vi "ble_wait_ms.vi"(6 "milliseconds to wait (100)":u32=100, 8 "error in (no error)":errorcluster) -> (0 "error out":errorcluster)   [LabVIEW 2017]
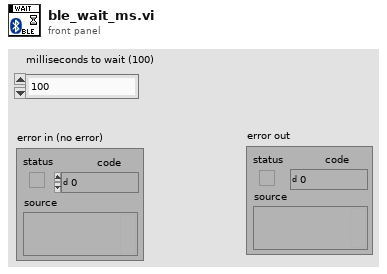
[diagram p1: front panel]
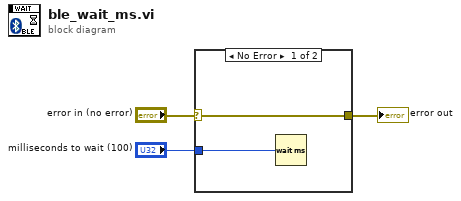
[diagram p0: block diagram]
diagram:
  n1 = case shown="No Error" "error in (no error)" {
    selector: "error in (no error)" -> [w5 w6]
    tunnel: [w5 w6] -> w2
    tunnel: "milliseconds to wait (100)" -> [w4 _]
    frame No Error {
      n2 = Wait (ms)(milliseconds to wait=w4) -> ()  [unwired: 1 out]
    }
    frame Error {
    }
  }
  "error out" <- w2
